vi "SpawnAsync.vi"(8 "ComponentActors":T1[](array[typedef]), 9 "PersistentActors":T1[](array[typedef]), 10 "MediatorAlias":string, 11 "Mediator":refnum<class "Actor.lvclass">) -> ()   [LabVIEW 2020, in "jettl.lvlib"]
uses:
  jettl.lvlib
  Actor/Actor.lvclass
  SpawnMediator.vi
  ActorMap.ctl
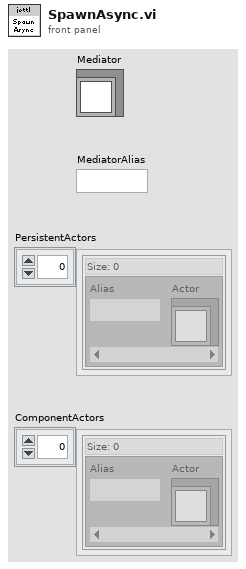
[diagram p1: front panel]
types:
  T1 = typedef "jettl.lvlib/ActorMap.ctl" = map{string, refnum<class "Actor.lvclass">}
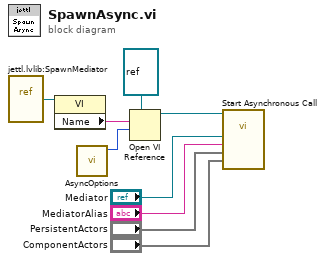
[diagram p0: block diagram]
diagram:
  n1 = vi-ref "jettl.lvlib:SpawnMediator.vi"() -> (w8:refnum<vi>)
  n2 = property class="VI"(reference=w8) -> ("Name"=w9:string)  [unwired: 1 in, 2 out]
  n3 = call "AsyncOptions.vi"() -> ("AsyncOptions"=w1:i32)  [unwired: 11 in]
  n4 = Open VI Reference(type specifier VI Refnum (for type only)=refnum<vi> refnum, vi path=w9, options=w1) -> (vi reference=w6:refnum<vi>)  [unwired: 3 in, 1 out]
  n5 = call-by-ref "Start Asynchronous Call"(reference=w6, "Components"="ComponentActors", "Persistent"="PersistentActors", "MediatorAlias"="MediatorAlias", "Mediator"="Mediator") -> ()  [unwired: 9 in, 2 out]
